vi "LRS Sums.vi"(9 "max":i32, 10 "i":i32, 11 "DataIn":i16) -> (3 "DataOut":T1)   [LabVIEW 2014]
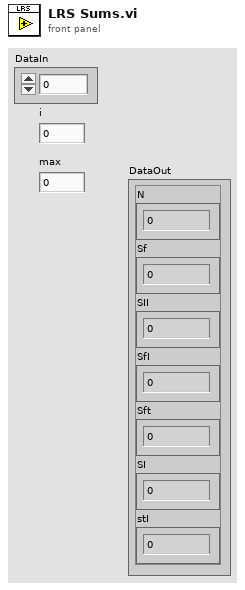
[diagram p1: front panel]
types:
  T1 = cluster{"N":i32, "Sf":fxp<+,54,54>, "SII":fxp<+,64,64>, "SfI":fxp<+,54,54>, "Sft":fxp<+,40,40>, "SI":fxp<+,54,54>, "stI":fxp<+,54,54>}
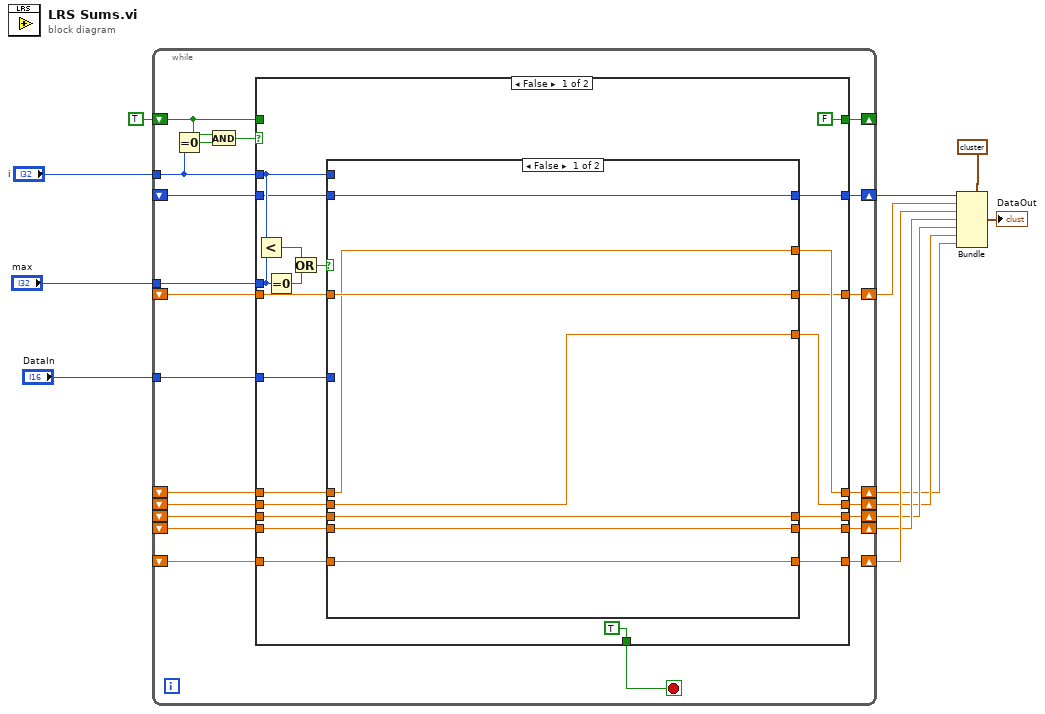
[diagram p0: block diagram]
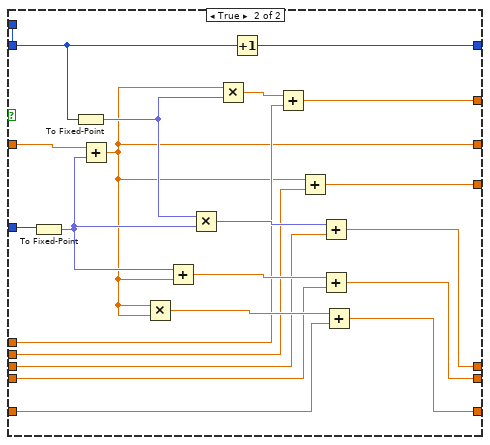
[diagram p2: hidden frame]
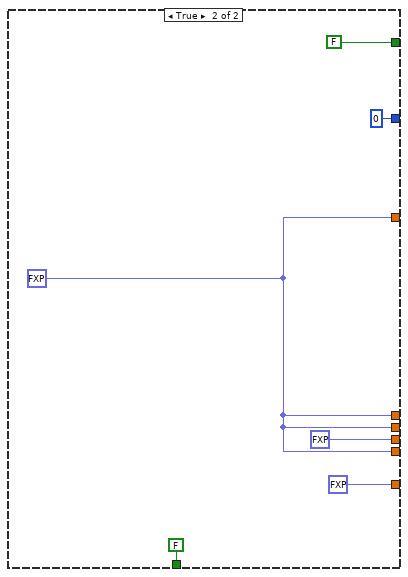
[diagram p3: hidden frame]
diagram:
  n1 = while {
    shift-right: [w35] -> w12
    shift-left: _ -> [w34]
    shift-right: [w33] -> w11
    shift-left: _ -> [w32]
    shift-right: [w21] -> w10
    shift-left: _ -> [w31]
    shift-right: [w30] -> w9
    shift-left: _ -> [w29]
    shift-right: [w28] -> w8
    shift-left: _ -> [w27]
    shift-right: [w26] -> w13
    shift-left: _ -> [w25]
    tunnel: "i" -> [w18]
    shift-right: [w23] -> w7
    shift-left: _ -> [w24]
    tunnel: "max" -> [w22]
    tunnel: "DataIn" -> [w20]
    shift-right: [w17] -> _
    shift-left: TRUE -> [w15]
    stop <- w19 stop-if-true
    n2 = Equal To 0?(x=w18) -> (x = 0?=w16:bool)
    n3 = And(x=w15, y=w16) -> (x .and. y?=w14:bool)
    n4 = case shown="False" w14 {
      tunnel: [w57 fxp<+,64,64> 0.0 ("fixed-point type")] -> w35
      tunnel: w34 -> [w56 _]
      tunnel: [w55 w87] -> w33
      tunnel: w32 -> [w54 _]
      tunnel: w31 -> [w53 _]
      tunnel: [w52 w87] -> w30
      tunnel: w29 -> [w51 _]
      tunnel: [w50 w87] -> w28
      tunnel: w27 -> [w49 _]
      tunnel: [w48 w87] -> w26
      tunnel: w25 -> [w47 _]
      tunnel: w18 -> [w44 _]
      tunnel: w24 -> [w42 _]
      tunnel: [w41 0] -> w23
      tunnel: w22 -> [w40 _]
      tunnel: [w39 fxp<+,40,40> 0.0 ("fixed-point type")] -> w21
      tunnel: w20 -> [w38 _]
      tunnel: [TRUE FALSE] -> w19
      tunnel: [FALSE FALSE] -> w17
      tunnel: w15 -> [_ _]
      frame False {
        n5 = Less?(x=w44, y=w40) -> (x < y?=w46:bool)
        n6 = Equal To 0?(x=w40) -> (x = 0?=w45:bool)
        n7 = Or(x=w46, y=w45) -> (x .or. y?=w43:bool)
        n8 = case shown="False" w43 {
          tunnel: [w58 w79] -> w57
          tunnel: w56 -> [w58 w78]
          tunnel: [w59 w77] -> w55
          tunnel: w54 -> [w59 w76]
          tunnel: [w60 w75] -> w39
          tunnel: w53 -> [w60 w74]
          tunnel: [w61 w73] -> w52
          tunnel: w51 -> [w61 w72]
          tunnel: [w62 w71] -> w50
          tunnel: w49 -> [w62 w70]
          tunnel: [w63 w69] -> w48
          tunnel: w47 -> [w63 w66]
          tunnel: w44 -> [_ w68]
          tunnel: w42 -> [w64 _]
          tunnel: [w64 w67] -> w41
          tunnel: w38 -> [_ w65]
          frame False {
          }
          frame True {
            n9 = To Fixed-Point(number=w65) -> (fixed-point=w84:fxp<+/-,16,16>)  [unwired: 1 in]
            n10 = To Fixed-Point(number=w68) -> (fixed-point=w83:fxp<+/-,32,32>)  [unwired: 1 in]
            n11 = Add(x=w66, y=w84) -> (x+y=w69:dbl)
            n12 = Multiply(x=w69, y=w69) -> (x*y=w80:dbl)
            n13 = Add(x=w84, y=w69) -> (x+y=w81:dbl)
            n14 = Multiply(x=w83, y=w84) -> (x*y=w82:fxp<+/-,48,48>)
            n15 = Multiply(x=w69, y=w83) -> (x*y=w85:dbl)
            n16 = Increment(x=w68) -> (x+1=w67:i32)
            n17 = Add(x=w85, y=w70) -> (x+y=w71:dbl)
            n18 = Add(x=w69, y=w72) -> (x+y=w73:dbl)
            n19 = Add(x=w82, y=w74) -> (x+y=w75:dbl)
            n20 = Add(x=w81, y=w76) -> (x+y=w77:dbl)
            n21 = Add(x=w80, y=w78) -> (x+y=w79:dbl)
          }
        }
      }
      frame True {
        w87 = fxp<+,54,54> 0.0
      }
    }
  }
  n22 = Bundle(cluster=T1 {"N"=0, "Sf"=0.0, "SII"=0.0, "SfI"=0.0, "Sft"=0.0, "SI"=0.0, "stI"=0.0} ("output cluster"), "N"=w7, "Sf"=w13, "SII"=w12, "SfI"=w11, "Sft"=w10, "SI"=w9, "stI"=w8) -> (→"DataOut":T1)
